vi "ui get all portrait files list.vi"() -> ()   [LabVIEW 2023]
panel:
  out "Files with error":i32
  out "Files with read error":path[](array[path])
  out "Progress":string
  out "size(s)":i32
  out "All Files in Dir":path[](array[path])
  in  "pattern (*.jpg)":string="*.jpg"
  in  "Folder Path":path
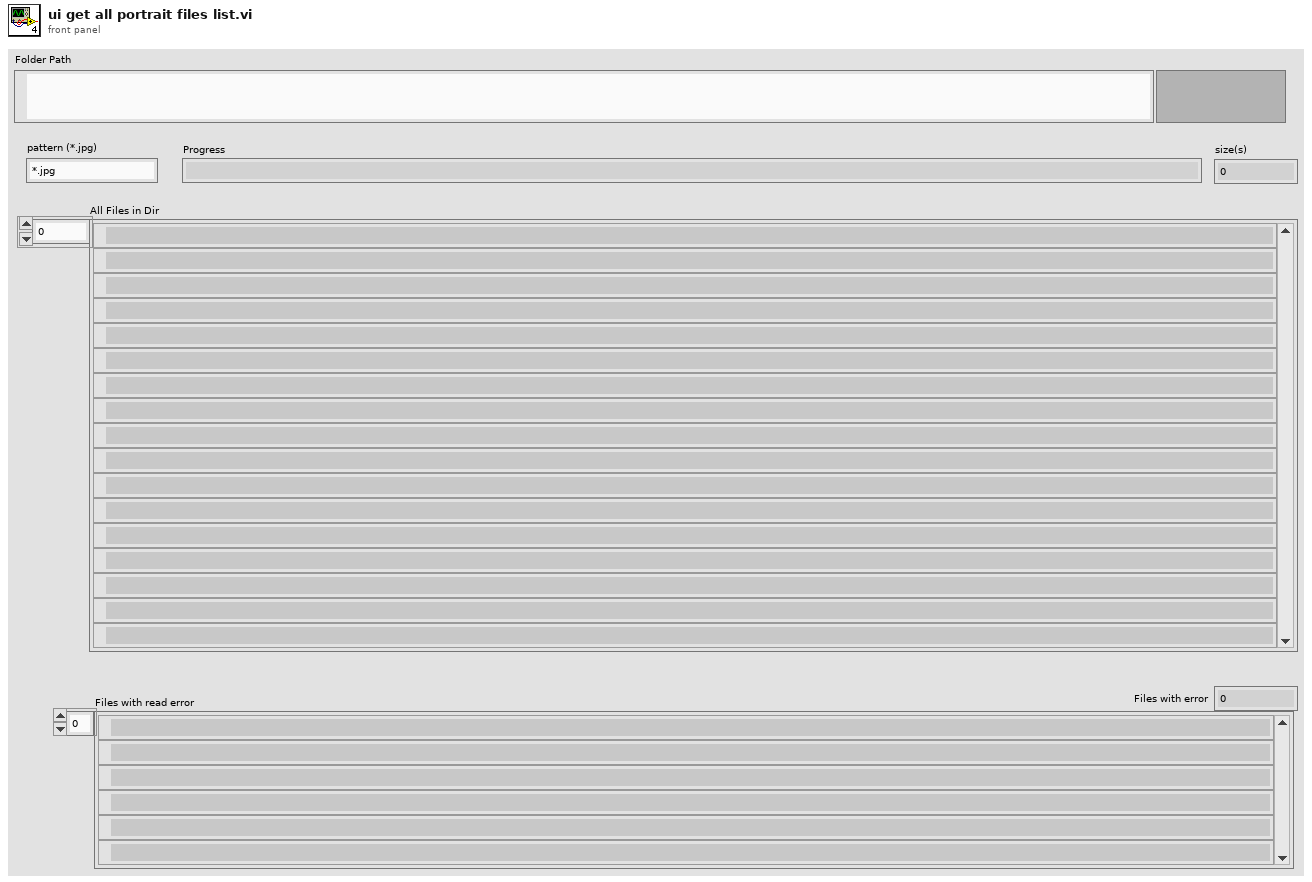
[diagram p1: front panel]
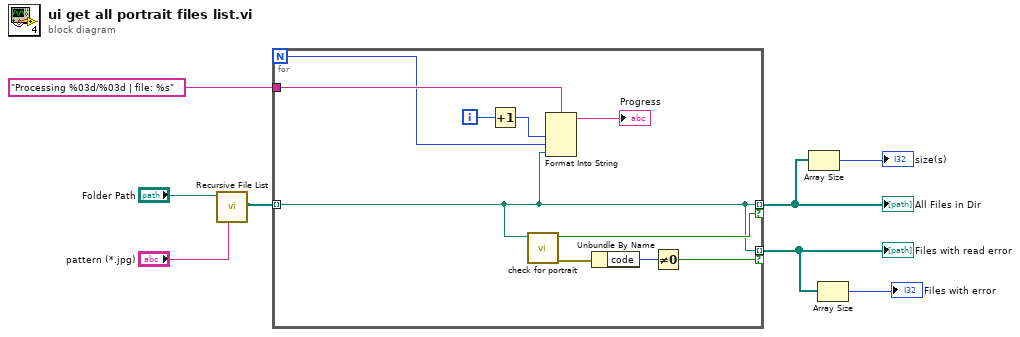
[diagram p0: block diagram]
diagram:
  n1 = call <vilib>:"Recursive File List.vi"("pattern"="pattern (*.jpg)", "Folder Path"="Folder Path") -> ("All Files in Dir"=w6:path[])  [unwired: 5 in, 4 out]
  n2 = for {
    N -> [w13]
    tunnel: w6 -> [w12] mode=indexing
    tunnel: [w12] -> w4 mode=indexing if=w18
    tunnel: "Processing %03d/%03d | file: %s" ("String") -> [w16]
    tunnel: [w12] -> w1 mode=indexing if=w11
    i -> [w15]
    n3 = Increment(x=w15) -> (x+1=w14:i32)
    n4 = call "check for portrait.vi"("path"=w12) -> ("error out"=w10:errorcluster, "Boolean"=w18:bool)  [unwired: 8 in, 1 out]
    n5 = Format Into String(format string=w16, w14, w13, w12) -> (resulting string=→"Progress":string)  [unwired: 2 in, 1 out]
    n6 = Unbundle By Name(w10) -> ("code"=w9:i32)
    n7 = Not Equal To 0?(x=w9) -> (x != 0?=w11:bool)
  }
  "All Files in Dir" <- w4
  "Files with read error" <- w1
  n8 = Array Size(array=w4) -> (size(s)=→"size(s)":i32)
  n9 = Array Size(array=w1) -> (size(s)=→"Files with error":i32)
